vi "exchangeData.vi"() -> ()   [LabVIEW 2015]
doc: "Dieses VI demonstriert, wie eine einfache TCP-Verbindung hergestellt wird und Daten an einen festgelegten Port gesendet werden. Nach dem Senden der Daten wird die Verbindung beendet. Das VI hält an, wenn die TCP-Verbindung unterbrochen wird.\n\nBei den gesendeten Daten handelt es sich um ein Array aus drei Signalverläufen.\n\n<B>Hinweis:</B> Es wird das VI \"Simple Data Client.vi\" benötigt, das sich in derselben Bibliothek befindet."
uses:
  <vilib>/Utility/error.llb/DialogType.ctl
  <vilib>/Analysis/NI_AALBase.lvlib
panel:
  in  "Data To MATLAB":string
  out "Data From MATLAB":string
  in  "Stopp Communication":bool
  in  "Port":u16=2057 caption="Port to Connect" min=1025 step=1
  in  "IP-Addresse":string="localhost" caption="IP-Adresse"
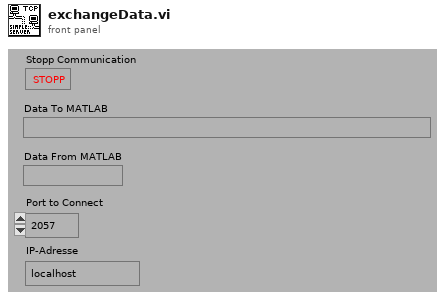
[diagram p1: front panel]
types:
  T1 = enum16{"Standard", "Buffered", "CRLF", "Immediate"}
  T2 = typedef "DialogType.ctl" = u16
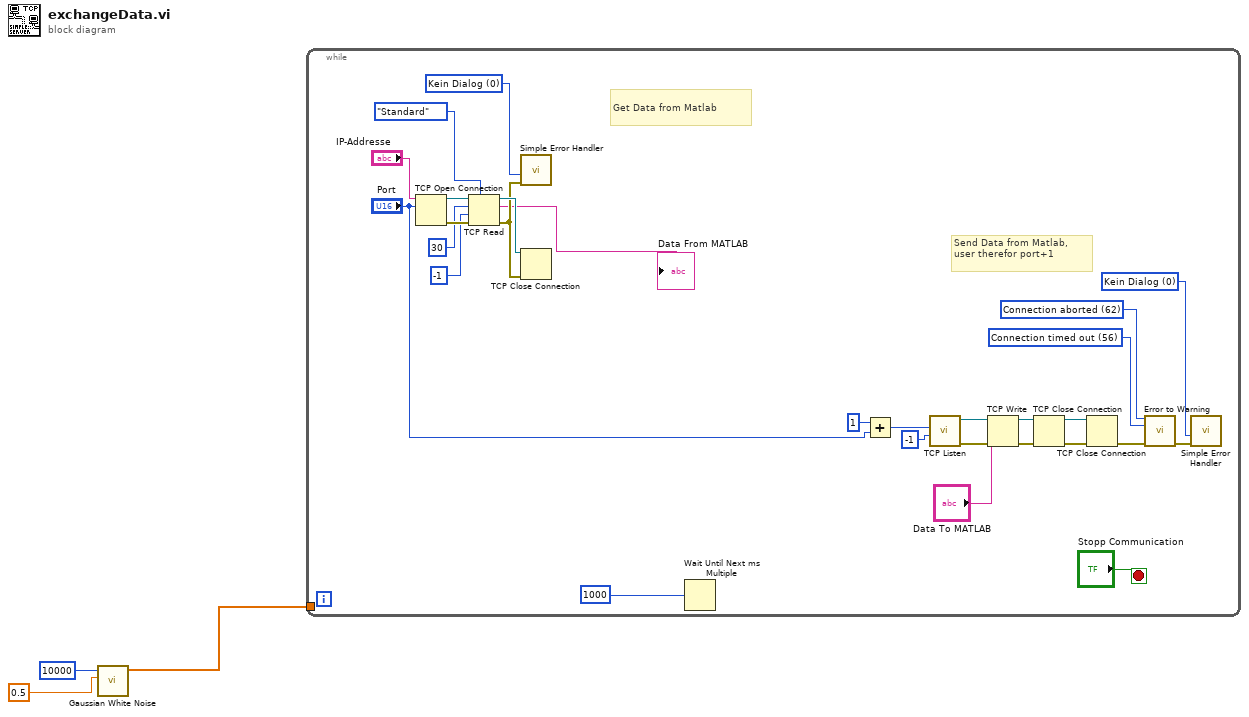
[diagram p0: block diagram]
diagram:
  n1 = call <vilib>:"Gaussian White Noise.vi"("standard deviation"=0.5 ("mean"), "samples"=10000 ("# of samples")) -> ("Gaussian noise pattern"=w3:dbl[])  [unwired: 8 in, 1 out]
  n2 = while {
    tunnel: w3 -> [_]
    stop <- "Stopp Communication" stop-if-true
    w7 = T2 0 items=["Kein Dialog", "OK-Meldung", "Dialog zum Fortsetzen oder Anhalten", "OK-Meldung + Warnungen", "Weiter/Stopp + Warnung"] ("type of dialog (OK msg:1)")
    w11 = 56 items=["No Error", "Argument Error", "Memory Full", "Out of Zone", "End of File", "File Already Open", "Generic File IO Error", "File Not Found", "File Permission Error", "Disk Full", "Duplicate Path", "Too Many Files Open", "Not Enabled", "Resource File Not Found", "Cannot Add Resource", "Resource Not Found", "Image Not Found", "Image Memory Error", "Pen Does Not Exist", "Config Bad Type", "Config Token Not Found", "Config Parse Error", "Config Memory Error", "Bad External Code Format", "Bad External Code Offset", "External Code Not Present", "Null Window", "Destroy Window Mixup", "Null Menu", "Print Aborted", "Bad Print Record", "Print Driver Error", "Windows Error During Print", "Memory Error During Print", "Print Dialog Error", "Generic Print Error", "Invalid Device Refnum", "Device Not Found", "Device Parameter Error", "Device Unit Error", "Can't Open Device", "Device Call Aborted", "Generic Error", "Cancelled By User", "Object ID Too Low", "Object ID Too High", "Object Not In Heap", "Unknown Heap", "Bad DefProc ID", "DefProc Not In Table", "Message Out Of Range", "Null Method", "Unknown Message", "Manager Call Not Supported", "Bad address", "Connection In progress", "Connection timed out", "Connection is already in progress", "Network attribute not supported", "Network error", "Address in use", "System out of memory", "Connection aborted", "Connection refused", "Connection is not connected", "Connection is already connected", "Connection closed", "Initialize error (interapplication manager)", "Bad occurrence", "Wait on unbound occurrence handler", "Occurrence queue overflow", "Bad path", "Semaphore not signaled", "Unrecognized type (interapplication manager)"] ("2nd Error to Convert")
    w12 = 62 items=["No Error", "Argument Error", "Memory Full", "Out of Zone", "End of File", "File Already Open", "Generic File IO Error", "File Not Found", "File Permission Error", "Disk Full", "Duplicate Path", "Too Many Files Open", "Not Enabled", "Resource File Not Found", "Cannot Add Resource", "Resource Not Found", "Image Not Found", "Image Memory Error", "Pen Does Not Exist", "Config Bad Type", "Config Token Not Found", "Config Parse Error", "Config Memory Error", "Bad External Code Format", "Bad External Code Offset", "External Code Not Present", "Null Window", "Destroy Window Mixup", "Null Menu", "Print Aborted", "Bad Print Record", "Print Driver Error", "Windows Error During Print", "Memory Error During Print", "Print Dialog Error", "Generic Print Error", "Invalid Device Refnum", "Device Not Found", "Device Parameter Error", "Device Unit Error", "Can't Open Device", "Device Call Aborted", "Generic Error", "Cancelled By User", "Object ID Too Low", "Object ID Too High", "Object Not In Heap", "Unknown Heap", "Bad DefProc ID", "DefProc Not In Table", "Message Out Of Range", "Null Method", "Unknown Message", "Manager Call Not Supported", "Bad address", "Connection In progress", "Connection timed out", "Connection is already in progress", "Network attribute not supported", "Network error", "Address in use", "System out of memory", "Connection aborted", "Connection refused", "Connection is not connected", "Connection is already connected", "Connection closed", "Initialize error (interapplication manager)", "Bad occurrence", "Wait on unbound occurrence handler", "Occurrence queue overflow", "Bad path", "Semaphore not signaled", "Unrecognized type (interapplication manager)"] ("1st Error to Convert")
    w24 = T2 0 items=["Kein Dialog", "OK-Meldung", "Dialog zum Fortsetzen oder Anhalten", "OK-Meldung + Warnungen", "Weiter/Stopp + Warnung"] ("type of dialog (OK msg:1)")
    # "Send Data from Matlab, user therefor port+1"
    # "Get Data from Matlab"
    n3 = TCP Open Connection(address="IP-Addresse", remote port or service name="Port") -> (connection ID=w30:refnum<k5>, error out=w29:errorcluster)  [unwired: 3 in]
    n4 = TCP Read(connection ID=w30, bytes to read=30 ("Zu lesende Bytes"), error in (no error)=w29, 7:T1."Standard" ("Modus (Standard)"), 9:-1 ("Timeout in ms (25000)")) -> (connection ID out=w28:refnum<k5>, data out=→"Data From MATLAB":string, error out=w27:errorcluster)
    n5 = call <vilib>:"Simple Error Handler.vi"("type of dialog (OK msg:1)"=w24, "error in (no error)"=w27) -> ()  [unwired: 3 in, 5 out]
    n6 = TCP Close Connection(connection ID=w28, error in (no error)=w27) -> ()  [unwired: 1 in, 2 out]
    n7 = Wait Until Next ms Multiple(millisecond multiple=u32 1000 ("Vielfache von ms")) -> ()  [unwired: 1 out]
    n8 = Add(x=u16 1, y="Port") -> (x+y=w19:u16)
    n9 = call <vilib>:"TCP Listen.vi"("timeout ms (wait forever: -1)"=-1, "port"=w19) -> ("error out"=w17:errorcluster, "connection ID"=w18:refnum<k5>)  [unwired: 5 in, 3 out]
    n10 = TCP Write(connection ID=w18, data in="Data To MATLAB", error in (no error)=w17) -> (connection ID out=w8:refnum<k5>, error out=w15:errorcluster)  [unwired: 1 in, 1 out]
    n11 = TCP Close Connection(connection ID=w8, error in (no error)=w15) -> (connection ID out=w10:refnum<k5>, error out=w9:errorcluster)  [unwired: 1 in]
    n12 = TCP Close Connection(connection ID=w10, error in (no error)=w9) -> (error out=w14:errorcluster)  [unwired: 1 in, 1 out]
    n13 = call <vilib>:"Error to Warning.vi"("1st Error to Convert"=w12, "2nd Error to Convert"=w11, "error in"=w14) -> ("warning out"=w13:errorcluster)  [unwired: 12 in]
    n14 = call <vilib>:"Simple Error Handler.vi"("type of dialog (OK msg:1)"=w7, "error in (no error)"=w13) -> ()  [unwired: 3 in, 5 out]
  }
